vi "VCS Activate Channel.vi"(0 "axis in":cluster{"keyHandle":u32, "nodeId":u16}={"keyHandle"=0, "nodeId"=1}, 2 "channelNumber":u8, 3 "recorded object":T1, 5 "error in (no error)":errorcluster) -> (14 "axis out":cluster{"keyHandle":u32, "nodeId":u16}={"keyHandle"=0, "nodeId"=1}, 19 "error out":errorcluster)   [LabVIEW 2018]
doc: "<B>VCS_ActivateChannel</B> connects object for data recording. Start with channel number one!"
uses:
  Resources/EposCmd.dll
  Resources/EposCmd64.dll
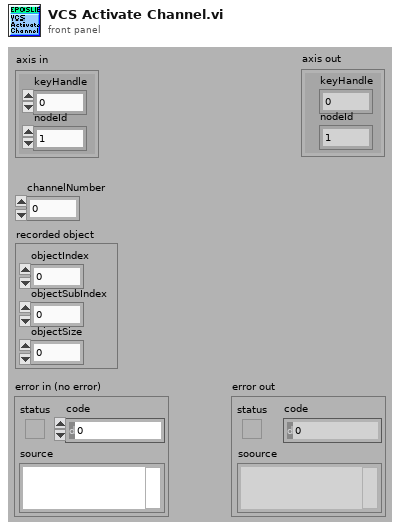
[diagram p1: front panel]
types:
  T1 = cluster{"objectIndex":u16, "objectSubIndex":u8, "objectSize":u8}
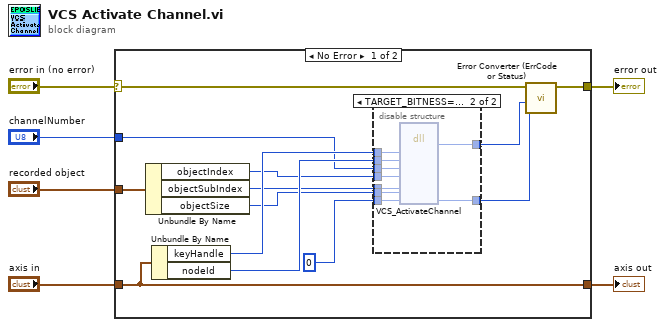
[diagram p0: block diagram]
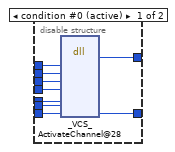
[diagram p2: hidden frame]
diagram:
  n1 = case shown="No Error" "error in (no error)" {
    selector: "error in (no error)" -> [w17 w38]
    tunnel: "axis in" -> [w19 w39]
    tunnel: [w19 w39] -> w5
    tunnel: [w18 w38] -> w4
    tunnel: "recorded object" -> [w11 _]
    tunnel: "channelNumber" -> [w7 _]
    frame No Error {
      n2 = Unbundle By Name(w11) -> ("objectIndex"=w10:u16, "objectSubIndex"=w9:u8, "objectSize"=w8:u8)
      n3 = Unbundle By Name(w19) -> ("keyHandle"=w13:u32, "nodeId"=w12:u16)
      n4 = disable-structure shown="TARGET_BITNESS==64" {
        disable-tunnel: [w28 w37] -> w16
        disable-tunnel: [w27 w36] -> w15
        disable-tunnel: u32 0 ("pErrorCode") -> [w26 w35]
        disable-tunnel: w13 -> [w25 w34]
        disable-tunnel: w12 -> [w24 w33]
        disable-tunnel: w10 -> [w23 w32]
        disable-tunnel: w9 -> [w22 w31]
        disable-tunnel: w8 -> [w21 w30]
        disable-tunnel: w7 -> [w20 w29]
        frame condition #0 (active) {
          n5 = dll-call lib="C:/Projeto em LabVIEW/EPOS-LabVIEW-Instrument-Driver-En/LabVIEW/maxon EPOS/Resources/EposCmd.*" fn="_VCS_ActivateChannel@28"("KeyHandle"=w25, "NodeId"=w24, "ChannelNumber"=w20, "ObjectIndex"=w23, "ObjectSubIndex"=w22, "ObjectSize"=w21, "pErrorCode"=w26) -> (w28:i32, "pErrorCode"=w27:u32)  [unwired: 9 in, 2 out]
        }
        frame condition #1 {
          n6 = dll-call lib="C:/setup/Resources/EposCmd64.*" fn="VCS_ActivateChannel" ("EposCmd.dll:_VCS_ActivateChannel@28")("KeyHandle"=w34, "NodeId"=w33, "ChannelNumber"=w29, "ObjectIndex"=w32, "ObjectSubIndex"=w31, "ObjectSize"=w30, "pErrorCode"=w35) -> ("Rückgabetyp"=w37:i32, "pErrorCode"=w36:u32)  [unwired: 9 in, 2 out]
        }
      }
      n7 = call "Error Converter (ErrCode or Status).vi"("error code"=w15, "return type"=w16, "error in (no error)"=w17) -> ("error out"=w18:errorcluster)  [unwired: 7 in]
    }
    frame Error {
    }
  }
  "error out" <- w4
  "axis out" <- w5
